vi "数据模拟实测.vi"() -> ()   [LabVIEW 2020]
uses:
  <vilib>/Utility/error.llb/DialogType.ctl
  <vilib>/Analysis/baseanly.llb/Mean (DBL).vi
  <vilib>/Utility/inputDevices.llb/mouseAcquire.vi
  <vilib>/Analysis/NI_AALBase.lvlib
panel:
  in  "退出":bool
  in  "选项卡控件":enum32{"数据文件界面", "实时模拟界面"}(tab)
  out "历史波形图":dbl[][](graph)
  out "数据采集起止时间":string
  in  "曲线标尺":bool[](array[boolean])=[TRUE, TRUE, TRUE, TRUE, TRUE, TRUE, TRUE, TRUE]
  in  "曲线隐显":bool[](array[boolean])=[TRUE, TRUE, TRUE, TRUE, TRUE, TRUE, TRUE, TRUE]
  in  "开始模拟":bool
  in  "重选文件":bool
  in  "刻棒选择":u16(ring) items=["D棒位"]
  in  "因子选择":i32(ring) items=["C1", "C2", "C3", "C4", "C5", "C6", "C7", "C8", "C9", "10"]
  in  "上段信号选择":i32(ring) items=["电流1", "电流2"]
  in  "下段信号选择":u16(ring)=1 items=["电流1", "电流2"]
  out "实时波形图":sgl[][](graph) caption="Waveform Chart - Dark"
  in  "曲线开关0":bool
  in  "曲线开关1":bool
  in  "曲线开关2":bool
  in  "曲线开关3":bool
  in  "曲线开关5":bool
  in  "曲线开关4":bool
  in  "自动调整Y标尺？":bool
  in  "自动/手动调整X标尺？":bool
  out "曲线0数字":dbl caption="电流1"
  out "曲线1数字":dbl caption="电流1反应性"
  out "曲线2数字":dbl caption="电流2"
  out "曲线3数字":dbl caption="电流2反应性"
  out "曲线4数字":dbl caption="D棒位"
  out "曲线5数字":dbl
  in  "仿真加速或减速倍数":dbl(slide)=0.1 min=-5.0 max=10.0 step=0.1 scale=-5.0..10.0 scale format="%#.1f"
  in  "备注说明":string
  out "上下段比值":dbl format="%0.2f"
  in  "合并DSF":bool
  in  "DRWM启用":bool
  in  "上段本底":dbl
  in  "下段本底":dbl
  in  "X标尺最小+":bool
  in  "X标尺最小-":bool
  in  "Y标尺最小+":bool
  in  "Y标尺最小-":bool
  in  "Y标尺最大+":bool
  in  "Y标尺最大-":bool
  out "AllStop":bool
  # "DRWM选项"
  # "DRWM控制"
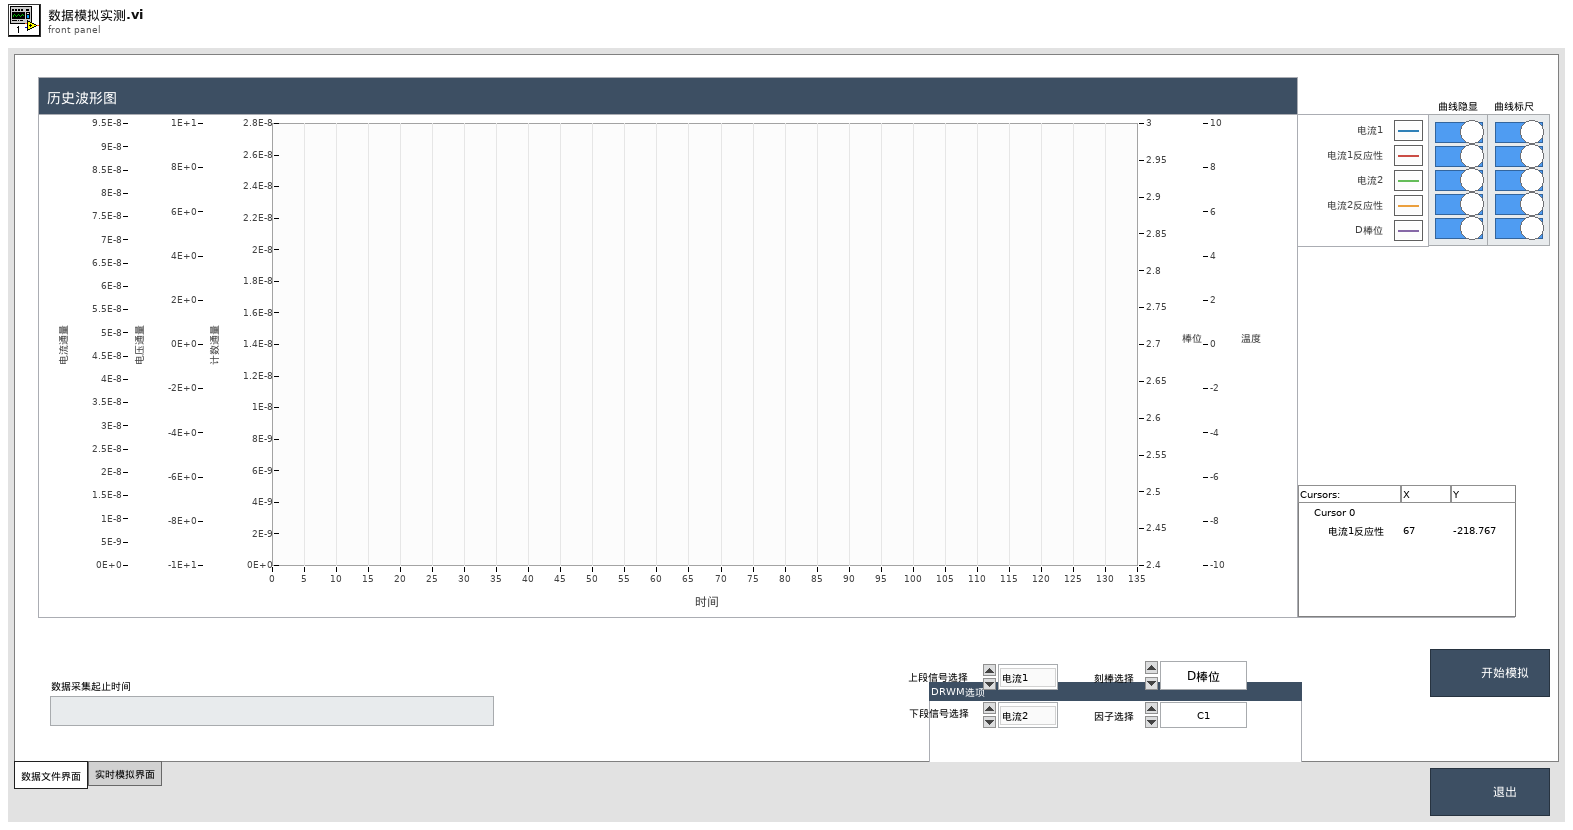
[diagram p1: front panel]
types:
  T1 = enum32{"Page Enabled", "Page Disabled", "Page Disabled & Grayed"}
  T2 = enum8{"Enabled", "Disabled", "Disabled and Grayed Out"}
  T3 = enum16{"open", "open or create", "create or replace", "create", "open (read only)"}
  T4 = typedef "DialogType.ctl" = u16
  T5 = cluster{"button 1":bool, "button 2":bool, "button 3":bool, "button 4":bool}
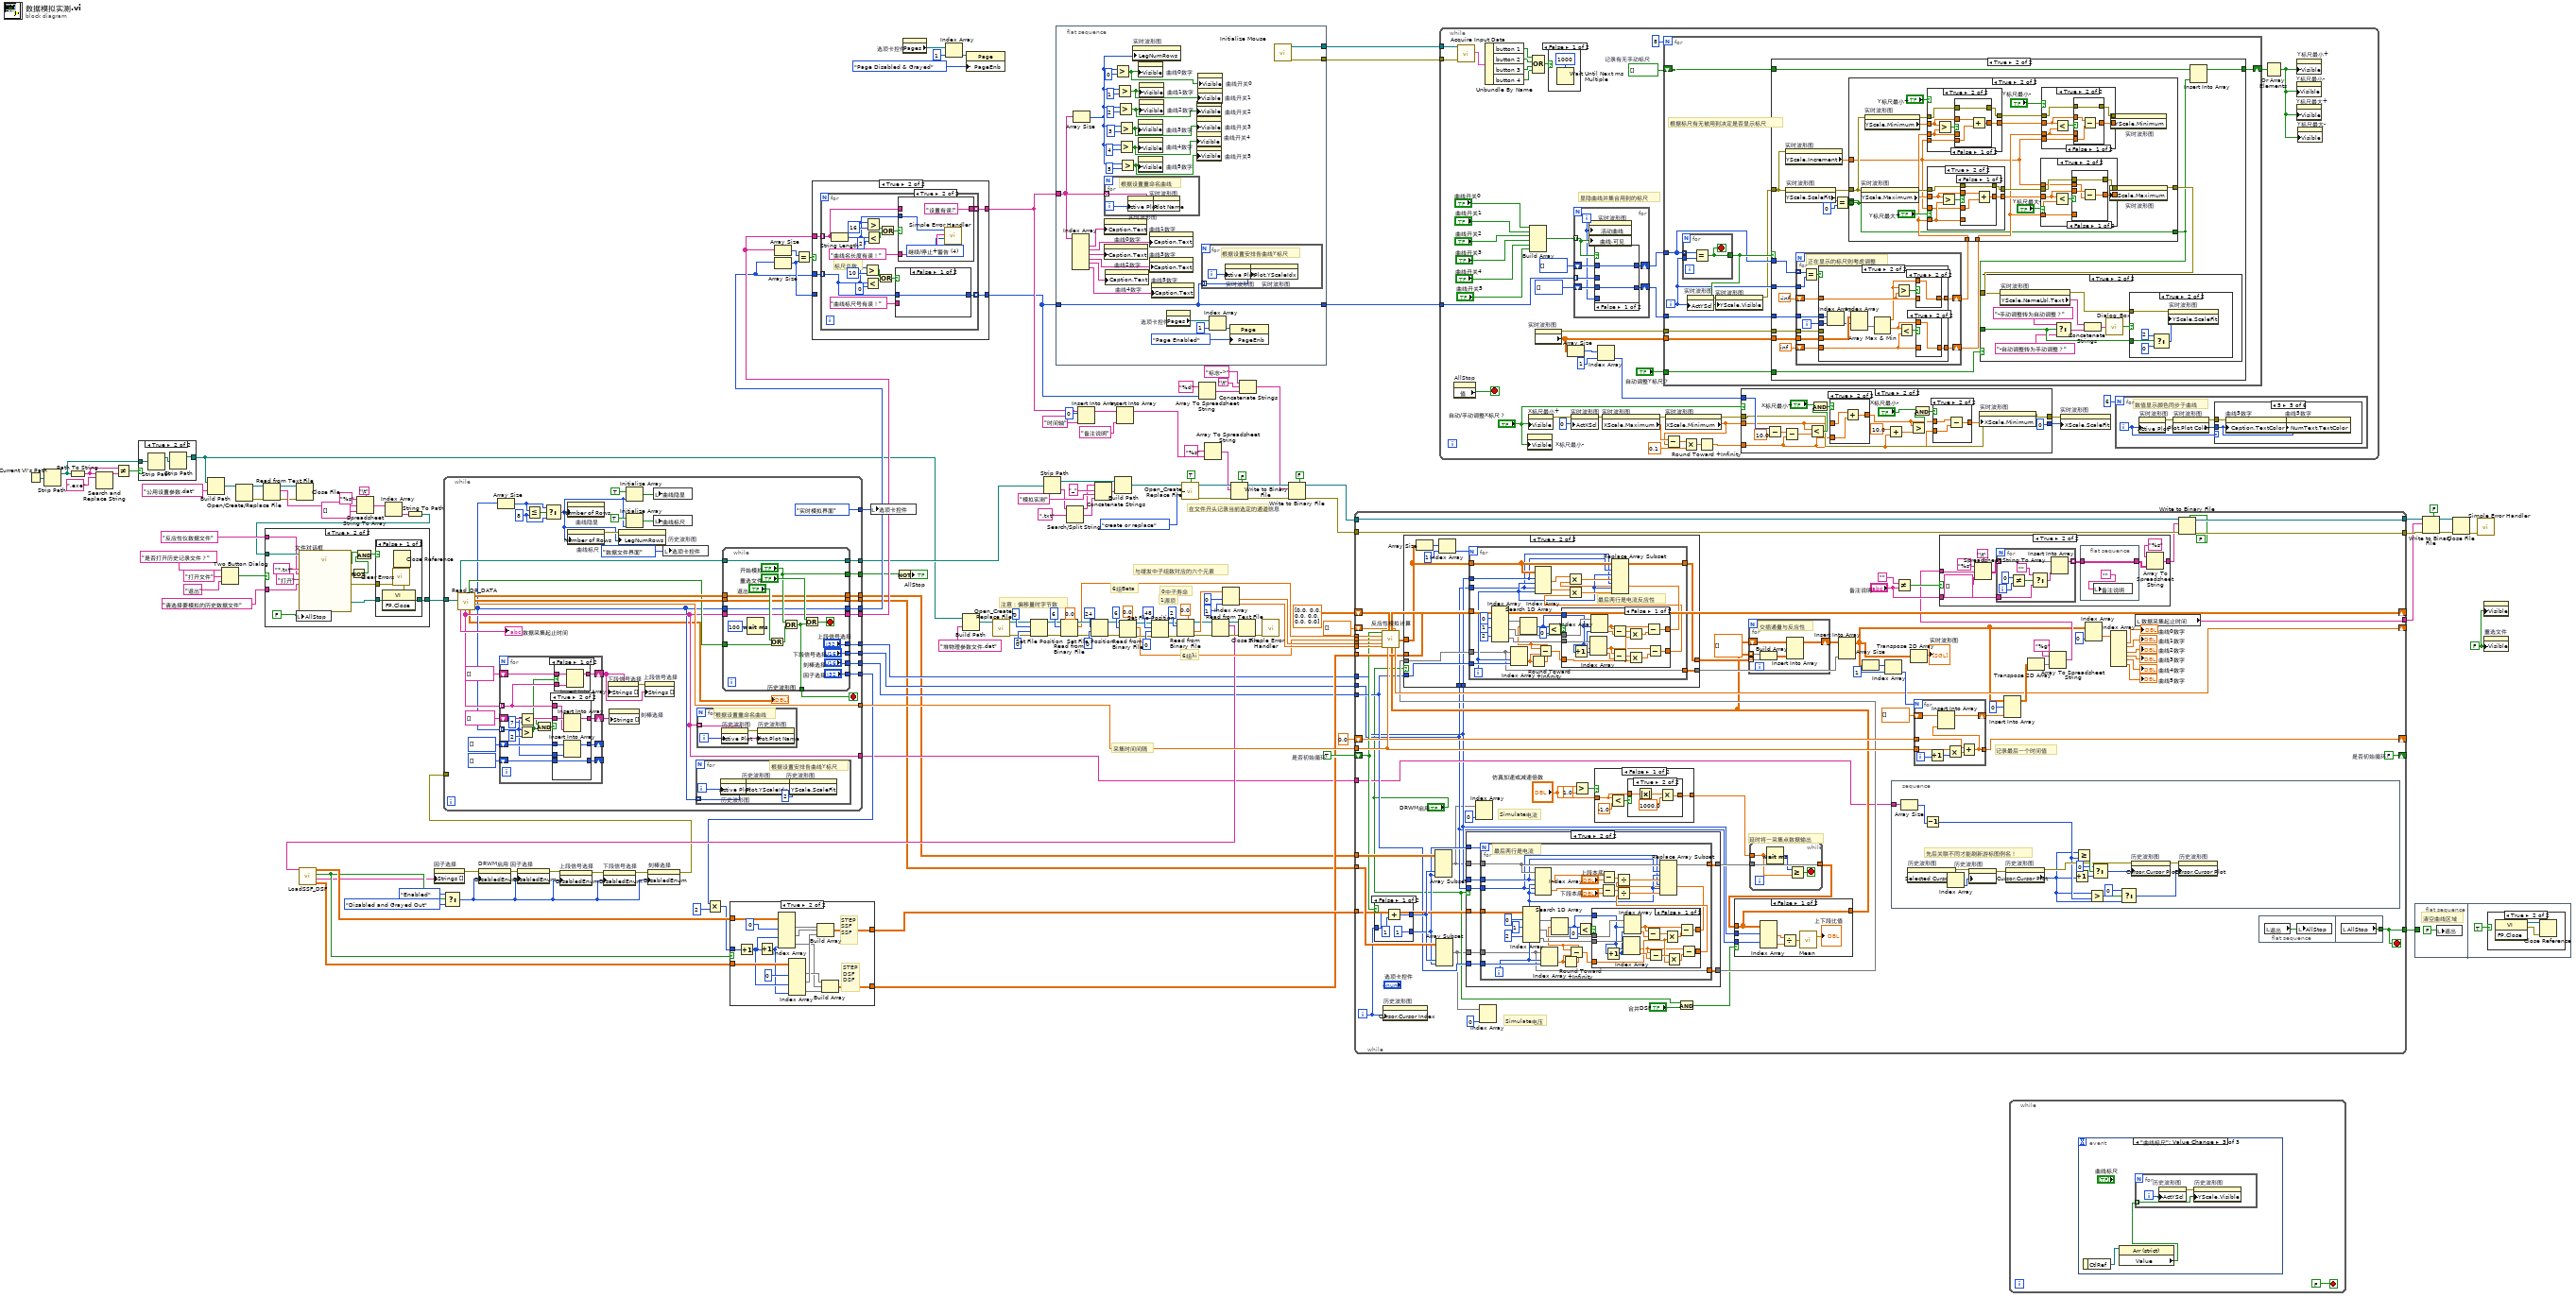
[diagram p0: block diagram]
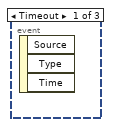
[diagram p2: hidden frame]
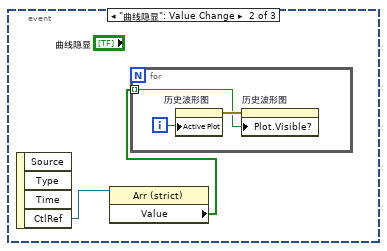
[diagram p3: hidden frame]
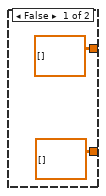
[diagram p4: hidden frame]
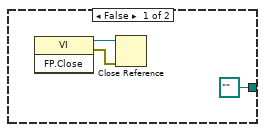
[diagram p5: hidden frame]
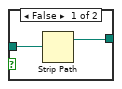
[diagram p7: hidden frame]
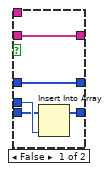
[diagram p9: hidden frame]
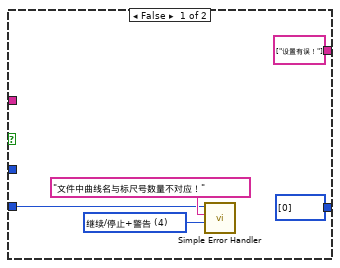
[diagram p11: hidden frame]
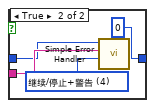
[diagram p12: hidden frame]
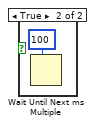
[diagram p14: hidden frame]
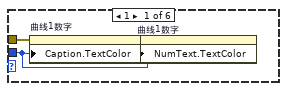
[diagram p15: hidden frame]
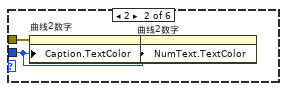
[diagram p16: hidden frame]
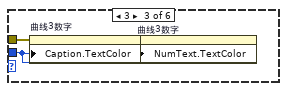
[diagram p17: hidden frame]
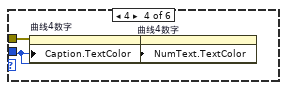
[diagram p18: hidden frame]
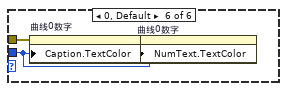
[diagram p19: hidden frame]
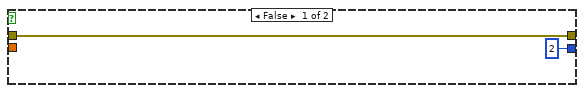
[diagram p20: hidden frame]
diagram:
  w5 = FALSE ("Visible")
  w122 = TRUE  # 是否初始循环
  # "6组λi"
  # "在文件开头记录当前选定的通道信息"
  # "采集时间间隔"
  # "注意：偏移量时字节数"
  # "与缓发中子组数对应的六个元素"
  # "0中子寿命"
  # "1源项"
  # "6组Beta"
  n1 = Current VI's Path() -> (path=w66:path)
  n2 = Strip Path(path=w66) -> (stripped path=w61:path)  [unwired: 1 out]
  n3 = Path To String(path=w61) -> (string=w63:string)
  n4 = Search and Replace String(input string=w63, search string=".exe" ("搜索字符串")) -> (result string=w64:string)  [unwired: 6 in, 3 out]
  n5 = Not Equal?(x=w63, y=w64) -> (x != y?=w62:bool)
  n6 = case shown="True" w62 {
    tunnel: w61 -> [w155 w158]
    tunnel: [w154 w156] -> w29
    frame False {
      n7 = Strip Path(path=w155) -> (stripped path=w154:path)  [unwired: 1 out]
    }
    frame True {
      n8 = Strip Path(path=w158) -> (stripped path=w157:path)  [unwired: 1 out]
      n9 = Strip Path(path=w157) -> (stripped path=w156:path)  [unwired: 1 out]
    }
  }
  n10 = Build Path(base path=w29, name or relative path="公用设置参数.dat") -> (appended path=w47:path)
  n11 = Two Button Dialog(message="是否打开历史记录文件？", 1:"退出" ("message"), 2:"打开文件" ("message")) -> (T button?=w57:bool)
  n12 = Open/Create/Replace File(file path (use dialog)=w47) -> (refnum out=w50:refnum<file>, error out=w51:errorcluster)  [unwired: 5 in, 1 out]
  n13 = Read from Text File(file (use dialog)=w50, error in=w51) -> (refnum out=w49:refnum<file>, text=w55:string, error out=w48:errorcluster)  [unwired: 1 in, 2 out]
  n14 = Close File(refnum=w49, error in=w48) -> ()  [unwired: 2 out]
  n15 = Spreadsheet String To Array(delimiter (Tab)="\t", format string="%s", spreadsheet string=w55, array type (2D Dbl)=string[] [] ("添加的数组")) -> (array=w56:string[])
  n16 = Index Array(array=w56) -> (element=w45:string)  [unwired: 1 in]
  n17 = String To Path(string=w45) -> (path=w58:path)
  n18 = case shown="True" w57 {
    tunnel: w58 -> [_ w174]
    tunnel: "请选择要模拟的历史数据文件" ("prompt") -> [_ w170]
    tunnel: "反应性仪数据文件" ("pattern label") -> [_ w169]
    tunnel: [path "" ("selected path") w167] -> w41
    frame False {
      n19 = invoke class="VI" method="FP.Close"() -> (reference out=w160:refnum<vi>, error out=w159:errorcluster)  [unwired: 3 in, 1 out]
      n20 = Close Reference(reference=w160, error in (no error)=w159) -> ()  [unwired: 1 out]
    }
    frame True {
      n21 = local write "AllStop"(FALSE ("退出程序")) -> ()
      n22 = call "文件对话框"("start path"=w174, "prompt"=w170, "button label"="打开", "pattern (all files)"="*.txt", "pattern label"=w169) -> ("selected path"=w168:path, "exists"=w165:bool, "cancelled"=w166:bool, "error out"=w162:errorcluster)  [unwired: 7 in]
      n23 = Not(x=w166) -> (.not. x?=w164:bool)
      n24 = And(x=w165, y=w164) -> (x .and. y?=w163:bool)
      n25 = case shown="False" w163 {
        tunnel: w168 -> [w178 w179]
        tunnel: [w178 w179] -> w167
        tunnel: w162 -> [w177 _]
        frame False {
          n26 = invoke class="VI" method="FP.Close"() -> (reference out=w175:refnum<vi>, error out=w176:errorcluster)  [unwired: 3 in, 1 out]
          n27 = call <vilib>:"Clear Errors.vi"("error in (no error)"=w177) -> ()  [unwired: 5 in, 2 out]
          n28 = Close Reference(reference=w175, error in (no error)=w176) -> ()  [unwired: 1 out]
        }
        frame True {
        }
      }
    }
  }
  n29 = property on="选项卡控件" class="TabCtl (strict)"() -> ("Pages"=w1:refnum<vi>[])  [unwired: 2 in, 2 out]
  n30 = Index Array(array=w1, index=1) -> (element=w2:refnum<vi>)
  n31 = Build Path(base path=w29, name or relative path="堆物理参数文件.dat" ("string")) -> (appended path=w134:path)
  n32 = property class="Page"(reference=w2, "PageEnb"=T1."Page Disabled & Grayed" ("Page Enabled State")) -> ()  [unwired: 1 in, 2 out]
  n33 = call <vilib>:"Open_Create_Replace File.vi"("file path"=w134) -> ("error out"=w118:errorcluster, "refnum"=w119:refnum<file>)  [unwired: 7 in, 2 out]
  n34 = Set File Position(offset (in bytes) (0)=0, refnum=w119, from (0:start)=0, error in=w118) -> (refnum out=w131:refnum<file>, error out=w130:errorcluster)
  n35 = flat-sequence {
    tunnel: w85 -> [w194]
    tunnel: [w184] -> w112
    tunnel: w84 -> [w184]
    tunnel: [w186] -> w121
    tunnel: [w185] -> w120
    frame #0 {
      n36 = Index Array(array=w194) -> (element #1=w206:string, element #2=w205:string, element #3=w204:string, element #4=w203:string, element #5=w202:string, element #6=w201:string)  [unwired: 6 in]
      n37 = Array Size(array=w194) -> (size(s)=w187:i32)
      n38 = property on="曲线0数字" class="DigNum (strict)"("Caption.Text"=w206) -> ()  [unwired: 2 in, 2 out]
      n39 = for {
        tunnel: w194 -> [w211] mode=indexing
        i -> [w212]
        # "根据设置重命名曲线"
        n40 = property on="实时波形图" class="WFChart (strict)"("Active Plot"=w212) -> (error out=w210:errorcluster)  [unwired: 2 in, 1 out]
        n41 = property on="实时波形图" class="WFChart (strict)"(error in=w210, "Plot.Plot Name"=w211) -> ()  [unwired: 1 in, 2 out]
      }
      n42 = property on="曲线2数字" class="DigNum (strict)"("Caption.Text"=w204) -> ()  [unwired: 2 in, 2 out]
      n43 = property on="曲线4数字" class="DigNum (strict)"("Caption.Text"=w202) -> ()  [unwired: 2 in, 2 out]
      n44 = Greater?(x=w187, y=0) -> (0:w193:bool)
      n45 = Greater?(x=w187, y=1) -> (0:w192:bool)
      n46 = Greater?(x=w187, y=2) -> (0:w191:bool)
      n47 = Greater?(x=w187, y=3) -> (0:w190:bool)
      n48 = Greater?(x=w187, y=4) -> (0:w189:bool)
      n49 = Greater?(x=w187, y=5) -> (0:w188:bool)
      n50 = property on="实时波形图" class="WFChart (strict)"("LegNumRows"=w187) -> ()  [unwired: 2 in, 2 out]
      n51 = property on="曲线0数字" class="DigNum (strict)"("Visible"=w193) -> ()  [unwired: 2 in, 2 out]
      n52 = property on="曲线3数字" class="DigNum (strict)"("Visible"=w190) -> ()  [unwired: 2 in, 2 out]
      n53 = property on="曲线4数字" class="DigNum (strict)"("Visible"=w189) -> ()  [unwired: 2 in, 2 out]
      n54 = property on="曲线5数字" class="DigNum (strict)"("Visible"=w188) -> ()  [unwired: 2 in, 2 out]
      n55 = property on="曲线1数字" class="DigNum (strict)"("Visible"=w192) -> ()  [unwired: 2 in, 2 out]
      n56 = property on="曲线2数字" class="DigNum (strict)"("Visible"=w191) -> ()  [unwired: 2 in, 2 out]
      n57 = property on="曲线1数字" class="DigNum (strict)"("Caption.Text"=w205) -> ()  [unwired: 2 in, 2 out]
      n58 = property on="曲线3数字" class="DigNum (strict)"("Caption.Text"=w203) -> ()  [unwired: 2 in, 2 out]
      n59 = property on="曲线5数字" class="DigNum (strict)"("Caption.Text"=w201) -> ()  [unwired: 2 in, 2 out]
      n60 = property on="选项卡控件" class="TabCtl (strict)"() -> ("Pages"=w183:refnum<vi>[])  [unwired: 2 in, 2 out]
      n61 = property on="曲线开关4" class="Bool (strict)"("Visible"=w189) -> ()  [unwired: 2 in, 2 out]
      n62 = property on="曲线开关2" class="Bool (strict)"("Visible"=w191) -> ()  [unwired: 2 in, 2 out]
      n63 = property on="曲线开关3" class="Bool (strict)"("Visible"=w190) -> ()  [unwired: 2 in, 2 out]
      n64 = property on="曲线开关5" class="Bool (strict)"("Visible"=w188) -> ()  [unwired: 2 in, 2 out]
      n65 = property on="曲线开关1" class="Bool (strict)"("Visible"=w192) -> ()  [unwired: 2 in, 2 out]
      n66 = property on="曲线开关0" class="Bool (strict)"("Visible"=w193) -> ()  [unwired: 2 in, 2 out]
      n67 = for {
        tunnel: w184 -> [w207] mode=indexing
        i -> [w209]
        # "根据设置安排各曲线Y标尺"
        n68 = property on="实时波形图" class="WFChart (strict)"("Active Plot"=w209) -> (error out=w208:errorcluster)  [unwired: 2 in, 1 out]
        n69 = property on="实时波形图" class="WFChart (strict)"(error in=w208, "Plot.YScaleIdx"=w207) -> ()  [unwired: 1 in, 2 out]
      }
      n70 = Index Array(array=w183, index=1) -> (element=w182:refnum<vi>)
      n71 = property class="Page"(reference=w182, "PageEnb"=T1."Page Enabled" ("Page Enabled State")) -> ()  [unwired: 1 in, 2 out]
      n72 = call <vilib>:"Initialize Mouse.vi"() -> ("error out"=w186:errorcluster, "device ID"=w185:refnum<k1>)  [unwired: 1 in, 9 out]
    }
  }
  n73 = Read from Binary File(5:sgl 0.0, 8:w130, 10:6, 11:w131) -> (0:w126:errorcluster, 2:w117:sgl[], 3:w127:refnum<file>)  [unwired: 2 in, 1 out]
  n74 = Set File Position(offset (in bytes) (0)=24, refnum=w127, from (0:start)=0, error in=w126) -> (refnum out=w129:refnum<file>, error out=w128:errorcluster)
  n75 = Read from Binary File(5:sgl 0.0, 8:w128, 10:6, 11:w129) -> (0:w124:errorcluster, 2:w75:sgl[], 3:w125:refnum<file>)  [unwired: 2 in, 1 out]
  n76 = Set File Position(offset (in bytes) (0)=48, refnum=w125, from (0:start)=0, error in=w124) -> (refnum out=w133:refnum<file>, error out=w132:errorcluster)
  n77 = Read from Binary File(5:sgl 0.0, 8:w132, 10:2, 11:w133) -> (0:w39:errorcluster, 2:w144:sgl[], 3:w40:refnum<file>)  [unwired: 2 in, 1 out]
  n78 = Read from Text File(file (use dialog)=w40, error in=w39) -> (refnum out=w38:refnum<file>, text=w36:string, error out=w37:errorcluster)  [unwired: 1 in, 2 out]
  n79 = call "LoadSSF_DSF.vi"("SF_PATH"=w36) -> ("下段因子数据"=w34:dbl[][], "因子棒号"=w25:string[], "SF_OK"=w28:bool, "上段因子数据"=w35:dbl[][])  [unwired: 6 in, 1 out]
  n80 = property on="因子选择" class="Ring (strict)"("Strings []"=w25) -> (error out=w24:errorcluster)  [unwired: 2 in, 1 out]
  n81 = Select(t=T2."Enabled" ("禁用"), s=w28, f=T2."Disabled and Grayed Out" ("禁用")) -> (s? t:f=w19:T2)
  n82 = property on="DRWM启用" class="Bool (strict)"(error in=w24, "DisabledEnum"=w19) -> (error out=w23:errorcluster)  [unwired: 1 in, 1 out]
  n83 = property on="因子选择" class="Ring (strict)"(error in=w23, "DisabledEnum"=w19) -> (error out=w21:errorcluster)  [unwired: 1 in, 1 out]
  n84 = property on="上段信号选择" class="Ring (strict)"(error in=w21, "DisabledEnum"=w19) -> (error out=w20:errorcluster)  [unwired: 1 in, 1 out]
  n85 = property on="下段信号选择" class="Ring (strict)"(error in=w20, "DisabledEnum"=w19) -> (error out=w18:errorcluster)  [unwired: 1 in, 1 out]
  n86 = property on="刻棒选择" class="Ring (strict)"(error in=w18, "DisabledEnum"=w19) -> (error out=w17:errorcluster)  [unwired: 1 in, 1 out]
  n87 = while {
    tunnel: [w249] -> w11
    tunnel: [w251] -> w69
    tunnel: [w250] -> w111
    tunnel: [w247] -> w110
    tunnel: [w248] -> w10
    tunnel: [w240] -> w108
    tunnel: [w245] -> w68
    tunnel: w41 -> [w244]
    tunnel: w17 -> [_]
    tunnel: [w237] -> w22
    tunnel: [w229] -> w14
    tunnel: [w228] -> w15
    tunnel: [w227] -> w16
    tunnel: [w226] -> w13
    tunnel: [enum32{"数据文件界面", "实时模拟界面"}."实时模拟界面" ("选项卡控件")] -> w12
    stop <- w246 stop-if-true
    w224 = 8 ("y")
    n88 = call "Read_DR_DATA.vi"("文件路径"=w244) -> ("标尺号"=w222:i32[], "时间步长"=w240:dbl, "P2数据"=w242:dbl[][], "通量数据"=w243:dbl[][], "曲线数据"=→"历史波形图":dbl[][], "读取正确?"=w241:bool, "曲线名称"=w226:string[], "数据采集起止时间"=→"数据采集起止时间":string, "filepath"=w239:path)  [unwired: 2 in]
    n89 = Array Size(array=w222) -> (size(s)=w223:i32)
    n90 = for {
      tunnel: w226 -> [w253] mode=indexing
      tunnel: w222 -> [w259] mode=indexing
      shift-right: [w265] -> w230
      shift-left: string[] [] -> [w266]
      shift-right: [w263] -> _
      shift-left: i32[] [] ("标尺号") -> [w264]
      shift-right: [w254] -> w231
      shift-left: string[] [] -> [w255]
      shift-right: [w261] -> _
      shift-left: i32[] [] ("标尺号") -> [w262]
      n91 = Greater?(x=w259, y=2) -> (0:w252:bool)
      n92 = Less?(x=w259, y=7) -> (x < y?=w257:bool)
      n93 = And(x=w257, y=w252) -> (x .and. y?=w256:bool)
      n94 = case shown="True" w256 {
        tunnel: w266 -> [w275 w282]
        tunnel: [w275 w281] -> w265
        tunnel: w264 -> [w274 w280]
        tunnel: [w274 w279] -> w263
        tunnel: w259 -> [w273 w278]
        tunnel: w253 -> [_ w277]
        tunnel: w262 -> [w272 w276]
        tunnel: [w271 w276] -> w261
        frame False {
          n95 = Insert Into Array(array=w272, new element=w273) -> (w271:i32[])  [unwired: 1 in]
        }
        frame True {
          n96 = Insert Into Array(array=w282, new element=w277) -> (w281:string[])  [unwired: 1 in]
          n97 = Insert Into Array(array=w280, new element=w278) -> (w279:i32[])  [unwired: 1 in]
        }
      }
      n98 = case shown="False" w252 {
        tunnel: w255 -> [w269 w270]
        tunnel: [w268 w270] -> w254
        tunnel: w253 -> [w267 _]
        frame False {
          n99 = Insert Into Array(array=w269, new element=w267) -> (w268:string[])  [unwired: 1 in]
        }
        frame True {
        }
      }
    }
    n100 = Less Or Equal?(x=w223, y=w224) -> (x <= y?=w225:bool)
    n101 = Select(t=w223, s=w225, f=w224) -> (s? t:f=w215:i32)
    n102 = property on="曲线隐显" class="Arr (strict)"("Number of Rows"=w215) -> ()  [unwired: 2 in, 2 out]
    n103 = property on="曲线标尺" class="Arr (strict)"("Number of Rows"=w215) -> (error out=w216:errorcluster)  [unwired: 2 in, 1 out]
    n104 = property on="下段信号选择" class="Ring (strict)"("Strings []"=w231) -> (error out=w232:errorcluster)  [unwired: 2 in, 1 out]
    n105 = property on="刻棒选择" class="Ring (strict)"("Strings []"=w230) -> ()  [unwired: 2 in, 2 out]
    n106 = property on="历史波形图" class="WFGraph (strict)"(error in=w216, "LegNumRows"=w215) -> ()  [unwired: 1 in, 2 out]
    n107 = Initialize Array(TRUE ("开始模拟"), w215) -> (w219:bool[])
    n108 = Initialize Array(TRUE ("开始模拟"), w215) -> (w218:bool[])
    n109 = property on="上段信号选择" class="Ring (strict)"(error in=w232, "Strings []"=w231) -> ()  [unwired: 1 in, 2 out]
    n110 = local write "曲线隐显"(w219) -> ()
    n111 = local write "曲线标尺"(w218) -> ()
    n112 = local write "选项卡控件"(enum32{"数据文件界面", "实时模拟界面"}."数据文件界面" ("选项卡控件")) -> ()
    n113 = for {
      tunnel: w222 -> [w285] mode=indexing
      i -> [w287]
      # "根据设置安排各曲线Y标尺"
      n114 = property on="历史波形图" class="WFGraph (strict)"("Active Plot"=w287) -> (error out=w286:errorcluster)  [unwired: 2 in, 1 out]
      n115 = property on="历史波形图" class="WFGraph (strict)"(error in=w286, "Plot.YScaleIdx"=w285) -> (error out=w284:errorcluster)  [unwired: 1 in, 1 out]
      n116 = property on="历史波形图" class="WFGraph (strict)"(error in=w284, "YScale.ScaleFit"=u8 2 ("Y标尺.标尺调节")) -> ()  [unwired: 1 in, 2 out]
    }
    n117 = for {
      tunnel: w226 -> [w289] mode=indexing
      i -> [w290]
      # "根据设置重命名曲线"
      n118 = property on="历史波形图" class="WFGraph (strict)"("Active Plot"=w290) -> (error out=w288:errorcluster)  [unwired: 2 in, 1 out]
      n119 = property on="历史波形图" class="WFGraph (strict)"(error in=w288, "Plot.Plot Name"=w289) -> ()  [unwired: 1 in, 2 out]
    }
    n120 = while {
      tunnel: [w299] -> w249
      tunnel: [w297] -> w250
      tunnel: w242 -> [w299]
      tunnel: w226 -> [w297]
      tunnel: [w305] -> w246
      tunnel: ["开始模拟"] -> w251
      tunnel: w241 -> [w302]
      tunnel: w243 -> [w300]
      tunnel: [w300] -> w248
      tunnel: w222 -> [w298]
      tunnel: [w298] -> w247
      tunnel: [w295] -> w245
      tunnel: w239 -> [w295]
      tunnel: ["因子选择"] -> w237
      tunnel: ["上段信号选择"] -> w229
      tunnel: ["下段信号选择"] -> w228
      tunnel: ["刻棒选择"] -> w227
      stop <- w296 stop-if-true
      n121 = Wait (ms)(milliseconds to wait=u32 100 ("等待时间（毫秒）")) -> ()  [unwired: 1 out]
      n122 = Or(x="退出", y=w302) -> (x .or. y?=w303:bool)
      n123 = Or(x="开始模拟", y=w303) -> (x .or. y?=w305:bool)
      n124 = Or(x="重选文件", y=w305) -> (x .or. y?=w296:bool)
    }
  }
  n125 = Multiply(x=w22, y=u16 2) -> (x*y=w32:i32)
  n126 = case shown="True" w28 {
    tunnel: w35 -> [_ w324]
    tunnel: w34 -> [_ w322]
    tunnel: w32 -> [_ w323]
    tunnel: [dbl[][] [] w315] -> w31
    tunnel: [dbl[][] [] w314] -> w30
    frame False {
    }
    frame True {
      # "STEP\nDSF\nDSF"
      # "STEP\nSSF\nSSF"
      n127 = Increment(x=w323) -> (x+1=w311:i32)
      n128 = Increment(x=w311) -> (x+1=w310:i32)
      n129 = Index Array(array=w324, index (col) #1=0 ("索引 (行)"), index (col) #2=w311, index (col) #3=w310) -> (element #1=w321:dbl[], element #2=w320:dbl[], element #3=w317:dbl[])  [unwired: 3 in]
      n130 = Index Array(array=w322, index (col) #1=0 ("索引 (行)"), index (col) #2=w311, index (col) #3=w310) -> (element #1=w318:dbl[], element #2=w319:dbl[], element #3=w316:dbl[])  [unwired: 3 in]
      n131 = Build Array(w321, w320, w319) -> (w315:dbl[][])
      n132 = Build Array(w318, w317, w316) -> (w314:dbl[][])
    }
  }
  n133 = Array Size(array=w111) -> (size(s)=w116:i32)
  n134 = Array Size(array=w110) -> (size(s)=w114:i32)
  n135 = Equal?(x=w116, y=w114) -> (x = y?=w115:bool)
  n136 = case shown="True" w115 {
    tunnel: w114 -> [w327 _]
    tunnel: w110 -> [_ w333]
    tunnel: w111 -> [_ w332]
    tunnel: [i32[] [0] w331] -> w84
    tunnel: [string[] ["设置有误！"] w330] -> w85
    frame False {
      w329 = T4 4 items=["无对话框", "确定信息", "继续或停止信息", "确定信息＋警告", "继续/停止+警告"] ("type of dialog (OK msg:1)")
      n137 = call <vilib>:"Simple Error Handler.vi"("error code (no error:0)"=w327, "error source (\" \")"="文件中曲线名与标尺号数量不对应！" ("error source (\" \")"), "type of dialog (OK msg:1)"=w329) -> ()  [unwired: 2 in, 5 out]
    }
    frame True {
      n138 = for {
        tunnel: w333 -> [w338] mode=indexing
        tunnel: w332 -> [w335] mode=indexing
        tunnel: [w336] -> w331 mode=indexing
        tunnel: [w334] -> w330 mode=indexing
        # "标尺总数"
        n139 = String Length(string=w335) -> (length=w340:i32)
        n140 = Greater?(x=w338, y=10) -> (0:w343:bool)
        n141 = Less?(x=w338, y=0) -> (x < y?=w342:bool)
        n142 = Greater?(x=w340, y=16) -> (0:w347:bool)
        n143 = Less?(x=w340, y=2) -> (x < y?=w348:bool)
        n144 = Or(x=w343, y=w342) -> (x .or. y?=w339:bool)
        n145 = Or(x=w347, y=w348) -> (x .or. y?=w346:bool)
        n146 = case shown="False" w339 {
          tunnel: "曲线标尺号有误！" ("error source (\" \")") -> [_ w355]
          tunnel: w338 -> [w351 w354]
          tunnel: [w351 0] -> w336
          frame False {
          }
          frame True {
            w353 = T4 4 items=["无对话框", "确定信息", "继续或停止信息", "确定信息＋警告", "继续/停止+警告"] ("type of dialog (OK msg:1)")
            n147 = call <vilib>:"Simple Error Handler.vi"("error code (no error:0)"=w354, "error source (\" \")"=w355, "type of dialog (OK msg:1)"=w353) -> ()  [unwired: 2 in, 5 out]
          }
        }
        n148 = case shown="True" w346 {
          tunnel: "曲线名长度有误！" ("error source (\" \")") -> [_ w360]
          tunnel: w340 -> [_ w359]
          tunnel: w335 -> [w356 _]
          tunnel: [w356 "设置有误!"] -> w334
          frame False {
          }
          frame True {
            w358 = T4 4 items=["无对话框", "确定信息", "继续或停止信息", "确定信息＋警告", "继续/停止+警告"] ("type of dialog (OK msg:1)")
            n149 = call <vilib>:"Simple Error Handler.vi"("error code (no error:0)"=w359, "error source (\" \")"=w360, "type of dialog (OK msg:1)"=w358) -> ()  [unwired: 2 in, 5 out]
          }
        }
      }
    }
  }
  n150 = local write "选项卡控件"(w12) -> ()
  n151 = Not(x=w69) -> (.not. x?=→"AllStop":bool)
  n152 = Strip Path(path=w68) -> (stripped path=w70:path, name=w9:string)
  n153 = Search/Split String(string=w9, search string/char (-)=".txt" ("搜索字符串/字符(-)")) -> (substring before match=w7:string, match + rest of string=w6:string)  [unwired: 1 in, 1 out]
  n154 = Insert Into Array(array=w85, index=0 ("索引"), new element="时间轴" ("新元素/子数组")) -> (w90:string[])
  n155 = Concatenate Strings ("连接字符串")(w7, "_" ("string"), "模拟实测" ("字符串"), w6) -> (w71:string)
  n156 = Build Path(base path=w70, name or relative path=w71) -> (appended path=w72:path)
  n157 = Insert Into Array(array=w90, new element="备注说明" ("新元素/子数组")) -> (w89:string[])  [unwired: 1 in]
  n158 = call <vilib>:"Open_Create_Replace File.vi"("advisory dialog? (display:T)"=TRUE, "function (open:0)"=T3."create or replace", "file path"=w72) -> ("error out"=w106:errorcluster, "refnum"=w103:refnum<file>)  [unwired: 5 in, 2 out]
  n159 = Array To Spreadsheet String(array=w84, 3:"%d" ("format string")) -> (spreadsheet string=w94:string)  [unwired: 1 in]
  n160 = Array To Spreadsheet String(array=w89, 3:"%s" ("format string")) -> (spreadsheet string=w101:string)  [unwired: 1 in]
  n161 = Index Array(array=w144, index #1=0, index #2=1) -> (element #1=w137:sgl, element #2=w136:sgl)
  n162 = Write to Binary File(file (use dialog)=w103, data=w101, error in=w106, 5:FALSE ("预置数组或字符串大小？(T)")) -> (refnum out=w96:refnum<file>, error out=w95:errorcluster)  [unwired: 2 in, 1 out]
  n163 = Close File(refnum=w38, error in=w37) -> (error out=w123:errorcluster)  [unwired: 1 out]
  n164 = Concatenate Strings("标志->" ("字符串"), "\t", w94) -> (w91:string)
  n165 = call <vilib>:"Simple Error Handler.vi"("error in (no error)"=w123) -> ()  [unwired: 4 in, 5 out]
  n166 = Write to Binary File(file (use dialog)=w96, data=w91, error in=w95, 5:FALSE ("预置数组或字符串大小？(T)")) -> (refnum out=w86:refnum<file>, error out=w87:errorcluster)  [unwired: 2 in, 1 out]
  n167 = while {
    shift-right: [w428] -> _
    shift-left: sgl[][] [[0.0], [0.0], [0.0], [0.0], [0.0], [0.0]] -> [w429]
    tunnel: w117 -> [w430]
    tunnel: w75 -> [w435]
    tunnel: w137 -> [w427]
    tunnel: w136 -> [w426]
    shift-right: [w434] -> _
    shift-left: w122 -> [w375]
    tunnel: w86 -> [w425]
    tunnel: w87 -> [w433]
    tunnel: [w361] -> w113
    tunnel: [w432] -> w79
    tunnel: w108 -> [w396]
    tunnel: [w424] -> w80
    tunnel: w10 -> [w408]
    tunnel: w11 -> [w407]
    tunnel: [w388] -> w74
    shift-right: [w393] -> _
    shift-left: 0.0 -> [w392]
    shift-right: [w389] -> _
    shift-left: sgl[] [] ("N(0)OUT") -> [w390]
    tunnel: w31 -> [w384]
    tunnel: w30 -> [w383]
    tunnel: w16 -> [w374]
    tunnel: w15 -> [w371]
    tunnel: w14 -> [w372]
    tunnel: w13 -> [w373]
    i -> [w376]
    stop <- w361 stop-if-true
    w434 = FALSE  # 是否初始循环
    # "Simulate电流"
    # "Simulate电压"
    # "记录最后一个时间值"
    # "延时将一采集点数据输出"
    n168 = case shown="False" w375 {
      tunnel: [w620 0 ("索引")] -> w405
      tunnel: [1 ("索引") 2 ("索引")] -> w381
      tunnel: w376 -> [w619 _]
      frame False {
        n169 = Add(x=w619, y=1) -> (x+y=w620:i32)
      }
      frame True {
      }
    }
    n170 = property on="历史波形图" class="WFGraph (strict)"("Cursor.Cursor Index"=w376) -> ()  [unwired: 2 in, 2 out]
    n171 = Array Subset(array=w408, index (col)=w405, length (col)=w381) -> (w367:dbl[][])  [unwired: 2 in]
    n172 = Array Subset(array=w407, index (col)=w405, length (col)=w381) -> (w366:dbl[][])  [unwired: 2 in]
    n173 = case shown="True" "DRWM启用" {
      tunnel: w367 -> [w528 w535]
      tunnel: [w528 w534] -> w387
      tunnel: w366 -> [w527 w537]
      tunnel: w384 -> [_ w536]
      tunnel: w381 -> [_ w533]
      tunnel: w374 -> [_ w532]
      tunnel: [w527 w531] -> w379
      tunnel: w372 -> [_ w530]
      tunnel: w371 -> [_ w529]
      frame False {
      }
      frame True {
        n174 = for {
          N: w533 -> [_]
          tunnel: w537 -> [w554]
          tunnel: w536 -> [w567]
          tunnel: w535 -> [w552]
          tunnel: [w556] -> w534
          tunnel: w532 -> [w566]
          tunnel: [w554] -> w531
          tunnel: w530 -> [w548]
          tunnel: w529 -> [w547]
          i -> [w555]
          # "最后两行是电流"
          n175 = Index Array(array=w567, index (row) #1=0 ("禁用的索引 (列)"), index (row) #2=1 ("索引 (列)"), index (row) #3=2 ("索引 (列)")) -> (element #1=w565:dbl[], element #2=w561:dbl[], element #3=w560:dbl[])  [unwired: 3 in]
          n176 = Index Array(array=w552, index (row) #1=w548, index (col) #1=w555, index (row) #2=w547, index (col) #2=w555) -> (element #1=w542:dbl, element #2=w540:dbl)
          n177 = Index Array(array=w554, index (row)=w555, index (col)=w566) -> (element=w551:dbl)
          n178 = Round Toward +Infinity(x=w551) -> (ceil(x): smallest int >= x=w550:dbl)
          n179 = Search 1D Array ("搜索一维数组")(1D array=w565, element=w550) -> (index of element=w562:i32)  [unwired: 1 in]
          n180 = Subtract(x=w550, y=w551) -> (x-y=w549:dbl)
          n181 = Less?(x=w562, y=0) -> (x < y?=w563:bool)
          n182 = case shown="False" w563 {
            tunnel: w562 -> [w580 _]
            tunnel: w561 -> [w582 _]
            tunnel: w560 -> [w581 _]
            tunnel: [w574 1.0] -> w553
            tunnel: [w570 1.0] -> w559
            tunnel: w549 -> [w571 _]
            frame False {
              n183 = Increment(x=w580) -> (x+1=w579:i32)
              n184 = Index Array(array=w581, index #1=w580, index #2=w579) -> (element #1=w568:dbl, element #2=w573:dbl)
              n185 = Index Array(array=w582, index #1=w580, index #2=w579) -> (element #1=w576:dbl, element #2=w578:dbl)
              n186 = Subtract(x=w576, y=w578) -> (x-y=w577:dbl)
              n187 = Subtract(x=w568, y=w573) -> (x-y=w572:dbl)
              n188 = Multiply(x=w577, y=w571) -> (x*y=w575:dbl)
              n189 = Multiply(x=w572, y=w571) -> (x*y=w569:dbl)
              n190 = Subtract(x=w576, y=w575) -> (x-y=w574:dbl)
              n191 = Subtract(x=w568, y=w569) -> (x-y=w570:dbl)
            }
            frame True {
              n192 = One Button Dialog(message="SSF文件棒位索引错误！" ("消息")) -> (true=w586:bool)  [unwired: 1 in]
              n193 = Stop(stop? (T)=w586) -> ()
            }
          }
          n194 = Subtract(x=w540, y="下段本底") -> (x-y=w541:dbl)
          n195 = Subtract(x=w542, y="上段本底") -> (x-y=w543:dbl)
          n196 = Divide(x=w543, y=w553) -> (x/y=w558:dbl)
          n197 = Divide(x=w541, y=w559) -> (x/y=w557:dbl)
          n198 = Replace Array Subset(array=w552, new element #1=w558, index (row) #1=w548, index (col) #1=w555, new element #2=w557, index (row) #2=w547, index (col) #2=w555) -> (w556:dbl[][])
        }
      }
    }
    n199 = Index Array(array=w367, index (col)=0 ("索引 (行)")) -> ()  [unwired: 1 in, 1 out]
    n200 = Index Array(array=w366, index (col)=0 ("索引 (行)")) -> ()  [unwired: 1 in, 1 out]
    n201 = Greater?(x="仿真加速或减速倍数", y=1.0) -> (0:w412:bool)
    n202 = case shown="False" w412 {
      tunnel: "仿真加速或减速倍数" -> [w624 w634]
      tunnel: [w625 w633] -> w410
      frame False {
        n203 = Less?(x=w624, y=-1.0) -> (x < y?=w626:bool)
        n204 = case shown="True" w626 {
          tunnel: [1000.0 w631] -> w625
          tunnel: w624 -> [_ w629]
          frame False {
          }
          frame True {
            n205 = Absolute Value(x=w629) -> (abs(x)=w630:dbl)
            n206 = Multiply(x=w630, y=1000.0) -> (x*y=w631:dbl)
          }
        }
      }
      frame True {
        n207 = Divide(x=u32 1000, y=w634) -> (x/y=w633:dbl)
      }
    }
    n208 = And(x="DRWM启用", y="合并DSF") -> (x .and. y?=w369:bool)
    n209 = while {
      tunnel: w387 -> [w639]
      tunnel: [w639] -> w378
      tunnel: w410 -> [w637]
      stop <- w636 stop-if-true
      n210 = Wait (ms)(milliseconds to wait=w637) -> (millisecond timer value=w638:u32)
      n211 = Greater Or Equal?(x=w638, y=w637) -> (x >= y?=w636:bool)
    }
    n212 = case shown="False" w369 {
      tunnel: w378 -> [w455 w468]
      tunnel: [w455 w467] -> w377
      tunnel: w372 -> [w454 w460]
      tunnel: w371 -> [w453 w461]
      frame False {
        n213 = Index Array(array=w455, index (row) #1=w454, index (row) #2=w453) -> (element #1=w459:dbl[], element #2=w458:dbl[])  [unwired: 2 in]
        n214 = Divide(x=w459, y=w458) -> (x/y=w457:dbl[])
        n215 = call-poly <vilib>:"Mean.vi"("X"=w457) -> ("mean"=→"上下段比值":dbl)  [unwired: 1 out]
      }
      frame True {
        n216 = local read "上下段比值"() -> (w465:dbl)
        n217 = Index Array(array=w468, index (row) #1=w460, index (row) #2=w461) -> (element #1=w466:dbl[], element #2=w463:dbl[])  [unwired: 2 in]
        n218 = Divide(x=w466, y=w465) -> (x/y=w464:dbl[])
        n219 = Add(x=w464, y=w463) -> (x+y=w462:dbl[])
        n220 = Replace Array Subset(array=w468, new element #1=w462, index (row) #1=w460, new element #2=w462, index (row) #2=w461) -> (w467:dbl[][])  [unwired: 2 in]
      }
    }
    n221 = call "反应性模拟计算.vi"("循环次数"=w375, "λi*Ci(0)"=w429, "N(0)IN"=w390, "βi"=w430, "λi"=w435, "中子寿命"=w427, "源项"=w426, "采集间隔"=w396, "中子注量率"=w377) -> ("λi*Ci(t)"=w428:sgl[][], "反应性OUT"=w386:sgl[][], "N(0)OUT"=w389:sgl[])  [unwired: 4 in]
    n222 = case shown="True" "DRWM启用" {
      tunnel: w386 -> [w470 w476]
      tunnel: [w470 w479] -> w385
      tunnel: w383 -> [_ w480]
      tunnel: w374 -> [_ w481]
      tunnel: w379 -> [w469 w478]
      tunnel: [w469 w477] -> w382
      tunnel: w372 -> [_ w472]
      tunnel: w371 -> [_ w471]
      frame False {
      }
      frame True {
        n223 = Array Size(array=w476) -> (size(s)=w475:i32[])
        n224 = Index Array(array=w475, index=1 ("索引")) -> (element=w473:i32)
        n225 = for {
          N: w473 -> [_]
          tunnel: w478 -> [w490]
          tunnel: w480 -> [w507]
          tunnel: w476 -> [w495]
          tunnel: [w492] -> w479
          tunnel: w481 -> [w506]
          tunnel: [w490] -> w477
          tunnel: w472 -> [w486]
          tunnel: w471 -> [w485]
          i -> [w491]
          # "最后两行是电流反应性"
          n226 = Index Array(array=w507, index (row) #1=0 ("禁用的索引 (列)"), index (row) #2=1 ("索引 (列)"), index (row) #3=2 ("索引 (列)")) -> (element #1=w505:dbl[], element #2=w501:dbl[], element #3=w500:dbl[])  [unwired: 3 in]
          n227 = Index Array(array=w490, index (row)=w491, index (col)=w506) -> (element=w488:dbl)
          n228 = Round Toward +Infinity(x=w488) -> (ceil(x): smallest int >= x=w489:dbl)
          n229 = Search 1D Array(1D array=w505, element=w489) -> (index of element=w502:i32)  [unwired: 1 in]
          n230 = Index Array(array=w495, index (row) #1=w486, index (col) #1=w491, index (row) #2=w485, index (col) #2=w491) -> (element #1=w499:sgl, element #2=w498:sgl)
          n231 = Subtract(x=w489, y=w488) -> (x-y=w487:dbl)
          n232 = Less?(x=w502, y=0) -> (x < y?=w503:bool)
          n233 = case shown="False" w503 {
            tunnel: w502 -> [w519 _]
            tunnel: w501 -> [w522 _]
            tunnel: w500 -> [w521 _]
            tunnel: [w509 1.0] -> w497
            tunnel: [w508 1.0] -> w496
            tunnel: w487 -> [w514 _]
            frame False {
              n234 = Increment(x=w519) -> (x+1=w520:i32)
              n235 = Index Array(array=w521, index #1=w519, index #2=w520) -> (element #1=w511:dbl, element #2=w517:dbl)
              n236 = Index Array(array=w522, index #1=w519, index #2=w520) -> (element #1=w512:dbl, element #2=w518:dbl)
              n237 = Subtract(x=w512, y=w518) -> (x-y=w516:dbl)
              n238 = Subtract(x=w511, y=w517) -> (x-y=w515:dbl)
              n239 = Multiply(x=w516, y=w514) -> (x*y=w513:dbl)
              n240 = Multiply(x=w515, y=w514) -> (x*y=w510:dbl)
              n241 = Subtract(x=w512, y=w513) -> (x-y=w509:dbl)
              n242 = Subtract(x=w511, y=w510) -> (x-y=w508:dbl)
            }
            frame True {
              n243 = One Button Dialog(message="SSF文件棒位索引错误！" ("消息")) -> (true=w526:bool)  [unwired: 1 in]
              n244 = Stop(stop? (T)=w526) -> ()
            }
          }
          n245 = Multiply(x=w499, y=w497) -> (x*y=w494:dbl)
          n246 = Multiply(x=w498, y=w496) -> (x*y=w493:dbl)
          n247 = Replace Array Subset(array=w495, new element #1=w494, index (row) #1=w486, index (col) #1=w491, new element #2=w493, index (row) #2=w485, index (col) #2=w491) -> (w492:sgl[][])
        }
      }
    }
    n248 = for {
      tunnel: w377 -> [w642] mode=indexing
      tunnel: w385 -> [w641] mode=indexing
      shift-right: [w643] -> w406
      shift-left: sgl[][] [] ("平滑掉数据") -> [w644]
      # "交插通量与反应性"
      n249 = Build Array(w642, w641) -> (w640:dbl[][])
      n250 = Insert Into Array(array=w644, new element=w640) -> (w643:sgl[][])  [unwired: 2 in]
    }
    n251 = Insert Into Array(array=w406, new element=w382) -> (w362:sgl[][])  [unwired: 2 in]
    n252 = Array Size(array=w362) -> (size(s)=w400:i32[])
    n253 = Index Array(array=w400, index=1 ("索引")) -> (element=w398:i32)
    n254 = stacked-sequence {
      tunnel: w373 -> [w445]
      frame #0 {
        # "先后关联不同才能刷新游标图例名！"
        n255 = Array Size(array=w445) -> (size(s)=w444:i32)
        n256 = property on="历史波形图" class="WFGraph (strict)"() -> (error out=w450:errorcluster, "Selected Cursors"=w452:u32[])  [unwired: 2 in, 1 out]
        n257 = Decrement(x=w444) -> (x-1=w439:i32)
        n258 = Index Array(array=w452) -> (element=w451:u32)  [unwired: 1 in]
        n259 = property on="历史波形图" class="WFGraph (strict)"(error in=w450, "Active Cursor"=w451) -> (error out=w449:errorcluster)  [unwired: 1 in, 1 out]
        n260 = property on="历史波形图" class="WFGraph (strict)"(error in=w449) -> (error out=w446:errorcluster, "Cursor.Cursor Plot"=w437:i32)  [unwired: 1 in, 1 out]
        n261 = Increment(x=w437) -> (x+1=w441:i32)
        n262 = Greater Or Equal?(x=w437, y=w439) -> (x >= y?=w448:bool)
        n263 = Greater?(x=w437, y=w439) -> (0:w440:bool)
        n264 = Select(t=0, s=w448, f=w441) -> (s? t:f=w443:i32)
        n265 = Select(t=0, s=w440, f=w437) -> (s? t:f=w438:i32)
        n266 = property on="历史波形图" class="WFGraph (strict)"(error in=w446, "Cursor.Cursor Plot"=w443) -> (error out=w447:errorcluster)  [unwired: 1 in, 1 out]
        n267 = property on="历史波形图" class="WFGraph (strict)"(error in=w447, "Cursor.Cursor Plot"=w438) -> ()  [unwired: 1 in, 2 out]
      }
    }
    n268 = Not Equal?(x="", y="备注说明") -> (x != y?=w404:bool)
    n269 = Transpose 2D Array(2D array=w362) -> (transposed array=→"实时波形图":sgl[][])
    n270 = for {
      N: w398 -> [_]
      tunnel: w392 -> [w592]
      tunnel: w396 -> [w594]
      shift-right: [w590] -> w395
      shift-left: sgl[] [] -> [w591]
      tunnel: [w589] -> w393
      i -> [w588]
      n271 = Increment(x=w588) -> (x+1=w587:i32)
      n272 = Multiply(x=w594, y=w587) -> (x*y=w593:dbl)
      n273 = Add(x=w592, y=w593) -> (x+y=w589:dbl)
      n274 = Insert Into Array(array=w591, new element=w589) -> (w590:sgl[])  [unwired: 1 in]
    }
    n275 = Insert Into Array ("数组插入")(array=w362, index (row)=0 ("索引 (行)"), new element=w395) -> (w394:sgl[][])  [unwired: 1 in]
    n276 = Transpose 2D Array(2D array=w394) -> (transposed array=w422:sgl[][])
    n277 = Array To Spreadsheet String(array=w422, 3:"%g" ("format string")) -> (spreadsheet string=w380:string)  [unwired: 1 in]
    n278 = case shown="True" w404 {
      tunnel: [w595 w596] -> w401
      tunnel: "备注说明" -> [_ w605]
      tunnel: w380 -> [w595 w600]
      frame False {
      }
      frame True {
        n279 = Spreadsheet String To Array(delimiter (Tab)="\t", format string="%s", spreadsheet string=w600, array type (2D Dbl)=string[][] [] ("添加的数组")) -> (array=w601:string[][])
        n280 = for {
          tunnel: w601 -> [w615] mode=indexing
          tunnel: [w614] -> w599 mode=indexing
          tunnel: w605 -> [w609]
          i -> [w613]
          n281 = Not Equal?(x=0 ("y"), y=w613) -> (x != y?=w611:bool)
          n282 = Select(t="", s=w611, f=w609) -> (s? t:f=w610:string)
          n283 = Insert Into Array(array=w615, new element=w610) -> (w614:string[])  [unwired: 1 in]
        }
        n284 = flat-sequence {
          tunnel: w599 -> [w606]
          tunnel: [w606] -> w597
          frame #0 {
            n285 = local write "备注说明"("") -> ()
          }
        }
        n286 = Array To Spreadsheet String(array=w597, 3:"%s" ("format string")) -> (spreadsheet string=w596:string)  [unwired: 1 in]
      }
    }
    n287 = Index Array(array=w362, index (col)=0 ("索引 (行)")) -> (element=w419:sgl[])  [unwired: 1 in]
    n288 = Index Array(array=w419) -> (element #1=→"曲线0数字":sgl, element #2=→"曲线1数字":sgl, element #3=→"曲线2数字":sgl, element #4=→"曲线3数字":sgl, element #5=→"曲线4数字":sgl, element #6=→"曲线5数字":sgl)  [unwired: 6 in]
    n289 = local read "数据采集起止时间"() -> (w388:string)
    n290 = Write to Binary File(file (use dialog)=w425, data=w401, error in=w433, 5:FALSE ("预置数组或字符串大小？(T)")) -> (refnum out=w424:refnum<file>, error out=w432:errorcluster)  [unwired: 2 in, 1 out]
    n291 = flat-sequence {
      tunnel: [w617] -> w361
      frame #0 {
        n292 = local read "退出"() -> (w616:bool)
        n293 = local write "AllStop"(w616) -> ()
      }
      frame #1 {
        n294 = local read "AllStop"() -> (w617:bool)
      }
    }
  }
  n295 = while {
    tunnel: w112 -> [w676]
    tunnel: w121 -> [w651]
    tunnel: w120 -> [w650]
    stop <- w690 stop-if-true
    w674 = bool[] []  # 记录有无手动标尺
    # "显隐曲线并集合用到的标尺"
    n296 = property on="AllStop" class="Bool (strict)"() -> ("值"=w690:bool)  [unwired: 2 in, 2 out]
    n297 = call-poly <vilib>:"Acquire Input Data.vi"("device ID"=w650, "error in (no error)"=w651) -> ("button info"=w652:T5)  [unwired: 1 in, 16 out]
    n298 = Unbundle By Name(w652) -> ("button 1"=w649:bool, "button 2"=w648:bool, "button 3"=w647:bool, "button 4"=w646:bool)
    n299 = property on="X标尺最小-" class="Bool"("Visible"="自动/手动调整X标尺？") -> ()  [unwired: 2 in, 2 out]
    n300 = property on="X标尺最小+" class="Bool"("Visible"="自动/手动调整X标尺？") -> (error out=w668:errorcluster)  [unwired: 2 in, 1 out]
    n301 = Build Array("曲线开关0", "曲线开关1", "曲线开关2", "曲线开关3", "曲线开关4", "曲线开关5") -> (w683:bool[])
    n302 = Compound Arithmetic op=OR(w649, w648, w647, w646) -> (w645:bool)
    n303 = property on="实时波形图" class="WFChart (strict)"() -> (error out=w677:errorcluster, "History Data"=w666:sgl[][])  [unwired: 2 in, 1 out]
    n304 = case shown="False" w645 {
      frame False {
        n305 = Wait Until Next ms Multiple(millisecond multiple=u32 1000) -> ()  [unwired: 1 out]
      }
      frame True {
        n306 = Wait Until Next ms Multiple(millisecond multiple=u32 100) -> ()  [unwired: 1 out]
      }
    }
    n307 = Array Size(array=w666) -> (size(s)=w665:i32[])
    n308 = property on="实时波形图" class="WFChart (strict)"(error in=w668, "ActXScl"=0 ("活动X标尺")) -> (error out=w662:errorcluster)  [unwired: 1 in, 1 out]
    n309 = for {
      tunnel: w683 -> [w913] mode=indexing
      tunnel: w676 -> [w911] mode=indexing
      shift-right: [w910] -> w680
      shift-left: i32[] [] ("添加的数组") -> [w912]
      shift-right: [w907] -> w678
      shift-left: i32[] [] ("添加的数组") -> [w909]
      i -> [w908]
      n310 = property on="实时波形图" class="WFChart (strict)"("活动曲线"=w908, "曲线.可见"=w913) -> ()  [unwired: 2 in, 2 out]
      n311 = case shown="False" w913 {
        tunnel: w912 -> [w915 w921]
        tunnel: w911 -> [_ w920]
        tunnel: [w915 w919] -> w910
        tunnel: w909 -> [w914 w918]
        tunnel: w908 -> [_ w917]
        tunnel: [w914 w916] -> w907
        frame False {
        }
        frame True {
          n312 = Insert Into Array(array=w918, new element=w917) -> (w916:i32[])  [unwired: 1 in]
          n313 = Insert Into Array(array=w921, new element=w920) -> (w919:i32[])  [unwired: 1 in]
        }
      }
    }
    n314 = Index Array(array=w665, index=1 ("索引")) -> (element=w663:i32)
    n315 = property on="实时波形图" class="WFChart (strict)"(error in=w662) -> (error out=w661:errorcluster, "XScale.Maximum"=w659:dbl)  [unwired: 1 in, 1 out]
    n316 = for {
      N: 8 -> [_]
      tunnel: w680 -> [w750]
      tunnel: w678 -> [w751]
      tunnel: w677 -> [w749]
      tunnel: w666 -> [w748]
      tunnel: "自动调整Y标尺？" -> [w746]
      shift-right: [w744] -> w673
      shift-left: w674 -> [w745]
      i -> [w752]
      # "根据标尺有无被用到决定是否显示标尺"
      n317 = for {
        tunnel: w750 -> [w906] mode=indexing
        tunnel: w752 -> [w905]
        tunnel: [w904] -> w753
        stop <- w904 stop-if-true
        n318 = Equal?(x=w906, y=w905) -> (x = y?=w904:bool)
      }
      n319 = property on="实时波形图" class="WFChart (strict)"("ActYScl"=w752) -> (error out=w754:errorcluster)  [unwired: 2 in, 1 out]
      n320 = property on="实时波形图" class="WFChart (strict)"(error in=w754, "YScale.Visible"=w753) -> (error out=w747:errorcluster)  [unwired: 1 in, 1 out]
      n321 = case shown="True" w753 {
        tunnel: w752 -> [_ w774]
        tunnel: w751 -> [_ w773]
        tunnel: w750 -> [_ w775]
        tunnel: w749 -> [_ w772]
        tunnel: w748 -> [_ w771]
        tunnel: w747 -> [_ w763]
        tunnel: w746 -> [_ w761]
        tunnel: w745 -> [w755 w758]
        tunnel: [w755 w757] -> w744
        frame False {
        }
        frame True {
          n322 = property on="实时波形图" class="WFChart (strict)"(error in=w763) -> ("YScale.Increment"=w762:dbl)  [unwired: 1 in, 2 out]
          n323 = property on="实时波形图" class="WFChart (strict)"(error in=w763) -> (error out=w765:errorcluster, "YScale.ScaleFit"=w768:u8)  [unwired: 1 in, 1 out]
          n324 = for {
            tunnel: w775 -> [w884] mode=indexing
            tunnel: w774 -> [w883]
            tunnel: w773 -> [w882]
            tunnel: w772 -> [w879]
            tunnel: w771 -> [w878]
            shift-right: [w875] -> w764
            shift-left: inf -> [w877]
            shift-right: [w874] -> w766
            shift-left: -inf -> [w876]
            i -> [w881]
            # "正在显示的标尺则考虑调整"
            n325 = Equal?(x=w884, y=w883) -> (x = y?=w880:bool)
            n326 = case shown="True" w880 {
              tunnel: w882 -> [_ w899]
              tunnel: w881 -> [_ w898]
              tunnel: w879 -> [_ _]
              tunnel: w878 -> [_ w897]
              tunnel: [w886 w890] -> w875
              tunnel: w877 -> [w886 w889]
              tunnel: w876 -> [w885 w893]
              tunnel: [w885 w892] -> w874
              frame False {
              }
              frame True {
                n327 = Index Array(array=w899, index=w898) -> (element=w896:i32)
                n328 = Index Array(array=w897, index (row)=w896) -> (element=w895:sgl[])  [unwired: 1 in]
                n329 = Array Max & Min(array=w895) -> (max value=w891:sgl, min value=w888:sgl)  [unwired: 2 out]
                n330 = Greater?(x=w891, y=w893) -> (0:w894:bool)
                n331 = Less?(x=w888, y=w889) -> (x < y?=w887:bool)
                n332 = case shown="True" w894 {
                  tunnel: w893 -> [w902 _]
                  tunnel: [w902 w903] -> w892
                  tunnel: w891 -> [_ w903]
                  frame False {
                  }
                  frame True {
                  }
                }
                n333 = case shown="True" w887 {
                  tunnel: w889 -> [w900 _]
                  tunnel: [w900 w901] -> w890
                  tunnel: w888 -> [_ w901]
                  frame False {
                  }
                  frame True {
                  }
                }
              }
            }
          }
          n334 = Equal?(x=w768, y=u8 0) -> (x = y?=w759:bool)
          n335 = case shown="True" w759 {
            selector: w759 -> [w791 _]
            tunnel: w766 -> [_ w802]
            tunnel: w765 -> [w790 w813]
            tunnel: w764 -> [_ w797]
            tunnel: w759 -> [_ _]
            tunnel: w762 -> [_ w794]
            tunnel: [w790 w793] -> w760
            tunnel: [w791 w792] -> w756
            tunnel: w759 -> [_ w792]
            frame False {
            }
            frame True {
              n336 = property on="实时波形图" class="WFChart (strict)"(error in=w813) -> (error out=w811:errorcluster, "YScale.Maximum"=w812:dbl)  [unwired: 1 in, 1 out]
              n337 = property on="实时波形图" class="WFChart (strict)"(error in=w813) -> (error out=w803:errorcluster, "YScale.Minimum"=w804:dbl)  [unwired: 1 in, 1 out]
              n338 = case shown="True" "Y标尺最小+" {
                tunnel: w802 -> [_ w837]
                tunnel: w804 -> [w829 w835]
                tunnel: w803 -> [w830 w834]
                tunnel: [w830 w833] -> w800
                tunnel: [w829 w832] -> w798
                tunnel: w794 -> [_ w831]
                frame False {
                }
                frame True {
                  n339 = Greater?(x=w835, y=w837) -> (0:w836:bool)
                  n340 = case shown="False" w836 {
                    tunnel: [w839 w843] -> w832
                    tunnel: w837 -> [_ w843]
                    tunnel: w835 -> [w840 _]
                    tunnel: w834 -> [w841 w842]
                    tunnel: [w841 w842] -> w833
                    tunnel: w831 -> [w838 _]
                    frame False {
                      n341 = Add(x=w840, y=w838) -> (x+y=w839:dbl)
                    }
                    frame True {
                    }
                  }
                }
              }
              n342 = case shown="True" "Y标尺最大+" {
                tunnel: w802 -> [_ w867]
                tunnel: w812 -> [w859 w865]
                tunnel: w811 -> [w860 w864]
                tunnel: [w860 w863] -> w808
                tunnel: [w859 w862] -> w807
                tunnel: w794 -> [_ w861]
                frame False {
                }
                frame True {
                  n343 = Greater?(x=w865, y=w867) -> (0:w866:bool)
                  n344 = case shown="False" w866 {
                    tunnel: [w869 w873] -> w862
                    tunnel: w867 -> [_ w873]
                    tunnel: w865 -> [w870 _]
                    tunnel: w864 -> [w871 w872]
                    tunnel: [w871 w872] -> w863
                    tunnel: w861 -> [w868 _]
                    frame False {
                      n345 = Add(x=w870, y=w868) -> (x+y=w869:dbl)
                    }
                    frame True {
                    }
                  }
                }
              }
              n346 = case shown="True" "Y标尺最大-" {
                tunnel: w797 -> [_ w852]
                tunnel: w807 -> [w845 w850]
                tunnel: w808 -> [w844 w849]
                tunnel: [w845 w848] -> w806
                tunnel: [w844 w847] -> w805
                tunnel: w794 -> [_ w846]
                frame False {
                }
                frame True {
                  n347 = Less?(x=w850, y=w852) -> (x < y?=w851:bool)
                  n348 = case shown="False" w851 {
                    tunnel: [w854 w858] -> w848
                    tunnel: w852 -> [_ w858]
                    tunnel: w850 -> [w855 _]
                    tunnel: w849 -> [w856 w857]
                    tunnel: [w856 w857] -> w847
                    tunnel: w846 -> [w853 _]
                    frame False {
                      n349 = Subtract(x=w855, y=w853) -> (x-y=w854:dbl)
                    }
                    frame True {
                    }
                  }
                }
              }
              n350 = case shown="True" "Y标尺最小-" {
                tunnel: w797 -> [_ w822]
                tunnel: w798 -> [w815 w820]
                tunnel: w800 -> [w814 w819]
                tunnel: [w815 w818] -> w795
                tunnel: [w814 w817] -> w796
                tunnel: w794 -> [_ w816]
                frame False {
                }
                frame True {
                  n351 = Less?(x=w820, y=w822) -> (x < y?=w821:bool)
                  n352 = case shown="False" w821 {
                    tunnel: [w824 w828] -> w818
                    tunnel: w822 -> [_ w828]
                    tunnel: w820 -> [w825 _]
                    tunnel: w819 -> [w826 w827]
                    tunnel: [w826 w827] -> w817
                    tunnel: w816 -> [w823 _]
                    frame False {
                      n353 = Subtract(x=w825, y=w823) -> (x-y=w824:dbl)
                    }
                    frame True {
                    }
                  }
                }
              }
              n354 = property on="实时波形图" class="WFChart (strict)"(error in=w805, "YScale.Maximum"=w806) -> (error out=w793:errorcluster)  [unwired: 1 in, 1 out]
              n355 = property on="实时波形图" class="WFChart (strict)"(error in=w796, "YScale.Minimum"=w795) -> ()  [unwired: 1 in, 2 out]
            }
          }
          n356 = case shown="True" w761 {
            tunnel: w760 -> [_ w781]
            tunnel: w756 -> [_ w779]
            frame False {
            }
            frame True {
              n357 = property on="实时波形图" class="WFChart (strict)"(error in=w781) -> (error out=w778:errorcluster, "YScale.NameLbl.Text"=w783:string)  [unwired: 1 in, 1 out]
              n358 = Select(t="-手动调整转为自动调整？" ("format string"), s=w779, f="-自动调整转为手动调整？" ("format string")) -> (s? t:f=w784:string)
              n359 = Concatenate Strings ("连接字符串")(w783, w784) -> (w782:string)
              n360 = call "Dialog_Box.vi"("提示信息"=w782) -> ("选择结果"=w780:bool)
              n361 = case shown="True" w780 {
                tunnel: w779 -> [_ w789]
                tunnel: w778 -> [_ w785]
                frame False {
                }
                frame True {
                  n362 = Select(t=u8 2 ("y"), s=w789, f=u8 0 ("y")) -> (s? t:f=w786:u8)
                  n363 = property on="实时波形图" class="WFChart (strict)"(error in=w785, "YScale.ScaleFit"=w786) -> ()  [unwired: 1 in, 2 out]
                }
              }
            }
          }
          n364 = Insert Into Array(array=w758, new element=w756) -> (w757:bool[])  [unwired: 1 in]
        }
      }
    }
    n365 = property on="实时波形图" class="WFChart (strict)"(error in=w661) -> (error out=w660:errorcluster, "XScale.Minimum"=w658:dbl)  [unwired: 1 in, 1 out]
    n366 = Subtract(x=w659, y=w658) -> (x-y=w657:dbl)
    n367 = Multiply(x=w657, y=0.1) -> (x*y=w655:dbl)
    n368 = Round Toward +Infinity(x=w655) -> (ceil(x): smallest int >= x=w654:dbl)
    n369 = case shown="True" "自动/手动调整X标尺？" {
      tunnel: [2 ("活动X标尺") 0 ("活动X标尺")] -> w669
      tunnel: [w715 w717] -> w667
      tunnel: w660 -> [w715 w728]
      tunnel: w663 -> [_ w733]
      tunnel: w658 -> [_ w727]
      tunnel: w654 -> [_ w719]
      frame False {
      }
      frame True {
        n370 = Subtract(x=w733, y=10.0) -> (x-y=w726:dbl)
        n371 = Subtract(x=w726, y=w719) -> (x-y=w725:dbl)
        n372 = Less?(x=w727, y=w725) -> (x < y?=w730:bool)
        n373 = And(x="X标尺最小+", y=w730) -> (x .and. y?=w732:bool)
        n374 = case shown="True" w732 {
          tunnel: w727 -> [w740 w743]
          tunnel: [w740 w742] -> w721
          tunnel: w719 -> [_ w741]
          frame False {
          }
          frame True {
            n375 = Add(x=w743, y=w741) -> (x+y=w742:dbl)
          }
        }
        n376 = Add(x=10.0, y=w719) -> (x+y=w718:dbl)
        n377 = Greater?(x=w721, y=w718) -> (0:w722:bool)
        n378 = And(x="X标尺最小-", y=w722) -> (x .and. y?=w724:bool)
        n379 = case shown="True" w724 {
          tunnel: w721 -> [w736 w739]
          tunnel: [w736 w738] -> w729
          tunnel: w719 -> [_ w737]
          frame False {
          }
          frame True {
            n380 = Subtract(x=w739, y=w737) -> (x-y=w738:dbl)
          }
        }
        n381 = property on="实时波形图" class="WFChart (strict)"(error in=w728, "XScale.Minimum"=w729) -> (error out=w717:errorcluster)  [unwired: 1 in, 1 out]
      }
    }
    n382 = property on="实时波形图" class="WFChart (strict)"(error in=w667, "XScale.ScaleFit"=w669) -> ()  [unwired: 1 in, 2 out]
    n383 = for {
      N: 6 -> [_]
      i -> [w693]
      # "数值显示颜色同步于曲线"
      n384 = property on="实时波形图" class="WFChart (strict)"("Active Plot"=w693) -> (error out=w696:errorcluster)  [unwired: 2 in, 1 out]
      n385 = property on="实时波形图" class="WFChart (strict)"(error in=w696) -> (error out=w695:errorcluster, "Plot.Plot Color"=w694:u32)  [unwired: 1 in, 1 out]
      n386 = case shown="5" w693 {
        tunnel: w695 -> [w698 w701 w704 w707 w710 w713]
        tunnel: w694 -> [w697 w700 w703 w706 w709 w712]
        frame 1 {
          n387 = property on="曲线1数字" class="DigNum (strict)"(error in=w698, "Caption.TextColor"=w697) -> (error out=w699:errorcluster)  [unwired: 1 in, 1 out]
          n388 = property on="曲线1数字" class="DigNum (strict)"(error in=w699, "NumText.TextColor"=w697) -> ()  [unwired: 1 in, 2 out]
        }
        frame 2 {
          n389 = property on="曲线2数字" class="DigNum (strict)"(error in=w701, "Caption.TextColor"=w700) -> (error out=w702:errorcluster)  [unwired: 1 in, 1 out]
          n390 = property on="曲线2数字" class="DigNum (strict)"(error in=w702, "NumText.TextColor"=w700) -> ()  [unwired: 1 in, 2 out]
        }
        frame 3 {
          n391 = property on="曲线3数字" class="DigNum (strict)"(error in=w704, "Caption.TextColor"=w703) -> (error out=w705:errorcluster)  [unwired: 1 in, 1 out]
          n392 = property on="曲线3数字" class="DigNum (strict)"(error in=w705, "NumText.TextColor"=w703) -> ()  [unwired: 1 in, 2 out]
        }
        frame 4 {
          n393 = property on="曲线4数字" class="DigNum (strict)"(error in=w707, "Caption.TextColor"=w706) -> (error out=w708:errorcluster)  [unwired: 1 in, 1 out]
          n394 = property on="曲线4数字" class="DigNum (strict)"(error in=w708, "NumText.TextColor"=w706) -> ()  [unwired: 1 in, 2 out]
        }
        frame 5 {
          n395 = property on="曲线5数字" class="DigNum (strict)"(error in=w710, "Caption.TextColor"=w709) -> (error out=w711:errorcluster)  [unwired: 1 in, 1 out]
          n396 = property on="曲线5数字" class="DigNum (strict)"(error in=w711, "NumText.TextColor"=w709) -> ()  [unwired: 1 in, 2 out]
        }
        frame 0, Default {
          n397 = property on="曲线0数字" class="DigNum (strict)"(error in=w713, "Caption.TextColor"=w712) -> (error out=w714:errorcluster)  [unwired: 1 in, 1 out]
          n398 = property on="曲线0数字" class="DigNum (strict)"(error in=w714, "NumText.TextColor"=w712) -> ()  [unwired: 1 in, 2 out]
        }
      }
    }
    n399 = Or Array Elements(Boolean array=w673) -> (logical OR=w672:bool)
    n400 = property on="Y标尺最小-" class="Bool"("Visible"=w672) -> ()  [unwired: 2 in, 2 out]
    n401 = property on="Y标尺最小+" class="Bool"("Visible"=w672) -> ()  [unwired: 2 in, 2 out]
    n402 = property on="Y标尺最大+" class="Bool"("Visible"=w672) -> ()  [unwired: 2 in, 2 out]
    n403 = property on="Y标尺最大-" class="Bool"("Visible"=w672) -> ()  [unwired: 2 in, 2 out]
  }
  n404 = while {
    stop <- FALSE stop-if-true
    n405 = event shown="[2] \"曲线标尺\": Value Change" {
      selector: _ -> [_ _ _]
      dyn-events: _ -> [_ _ _]
      timeout: _ -> [_ _ _]
      event Timeout {
        n406 = event-data() -> ()  [unwired: 1 in, 3 out]
      }
      event "曲线隐显": Value Change {
        n407 = event-data() -> ("CtlRef"=w924:refnum<vi>)  [unwired: 1 in, 3 out]
        n408 = property class="Arr (strict)"(reference=w924) -> ("Value"=w923:bool[])  [unwired: 1 in, 2 out]
        n409 = for {
          tunnel: w923 -> [w925] mode=indexing
          i -> [w926]
          n410 = property on="历史波形图" class="WFGraph (strict)"("Active Plot"=w926) -> (error out=w927:errorcluster)  [unwired: 2 in, 1 out]
          n411 = property on="历史波形图" class="WFGraph (strict)"(error in=w927, "Plot.Visible?"=w925) -> ()  [unwired: 1 in, 2 out]
        }
      }
      event "曲线标尺": Value Change {
        n412 = event-data() -> ("CtlRef"=w929:refnum<vi>)  [unwired: 1 in]
        n413 = property class="Arr (strict)"(reference=w929) -> ("Value"=w928:bool[])  [unwired: 1 in, 2 out]
        n414 = for {
          tunnel: w928 -> [w931] mode=indexing
          i -> [w932]
          n415 = property on="历史波形图" class="WFGraph (strict)"("ActYScl"=w932) -> (error out=w930:errorcluster)  [unwired: 2 in, 1 out]
          n416 = property on="历史波形图" class="WFGraph (strict)"(error in=w930, "YScale.Visible"=w931) -> ()  [unwired: 1 in, 2 out]
        }
      }
    }
  }
  n417 = flat-sequence {
    tunnel: w113 -> [_]
    frame #0 {
      # "清空曲线区域"
      n418 = local write "退出"(FALSE ("取消")) -> ()
    }
    frame #1 {
      n419 = case shown="True" TRUE {
        frame False {
        }
        frame True {
          n420 = invoke class="VI" method="FP.Close"() -> (reference out=w935:refnum<vi>, error out=w936:errorcluster)  [unwired: 3 in, 1 out]
          n421 = Close Reference(reference=w935, error in (no error)=w936) -> ()  [unwired: 1 out]
        }
      }
    }
  }
  n422 = Write to Binary File(file (use dialog)=w80, data=w74, error in=w79, 5:FALSE ("预置数组或字符串大小？(T)")) -> (refnum out=w82:refnum<file>, error out=w81:errorcluster)  [unwired: 2 in, 1 out]
  n423 = Close File(refnum=w82, error in=w81) -> (error out=w83:errorcluster)  [unwired: 1 out]
  n424 = call <vilib>:"Simple Error Handler.vi"("error in (no error)"=w83) -> ()  [unwired: 4 in, 5 out]
  n425 = property class="Clust (strict)"("Visible"=w5) -> ()  [unwired: 2 in, 2 out]
  n426 = property on="重选文件" class="Bool"("Visible"=w5) -> ()  [unwired: 2 in, 2 out]
